vi "24-09-2020.vi"() -> ()   [LabVIEW 2020]
uses:
  <vilib>/measure/NI_MABase.lvlib
panel:
  out "reversed array":dbl[](array[numeric])
  in  "Numeric 4":dbl format="%#_13g"
  out "H":dbl
  out "D":dbl
  out "U":dbl
  in  "Numeric 3":dbl format="%#_13g"
  out "Waveform Graph 3":waveform(dbl)(graph)
  out "Numeric 2":i32
  out "numeric array":i16[](array[numeric])
  in  "Search Item":string
  in  "String":string
  in  "stop":bool
  out "Waveform Chart":dbl(graph)
  in  "Speed":dbl(slide) scale=0.0..10.0
  out "Waveform Graph 2":i32[](graph)
  out "Numeric":i32
  out "Waveform Graph":i32[](graph)
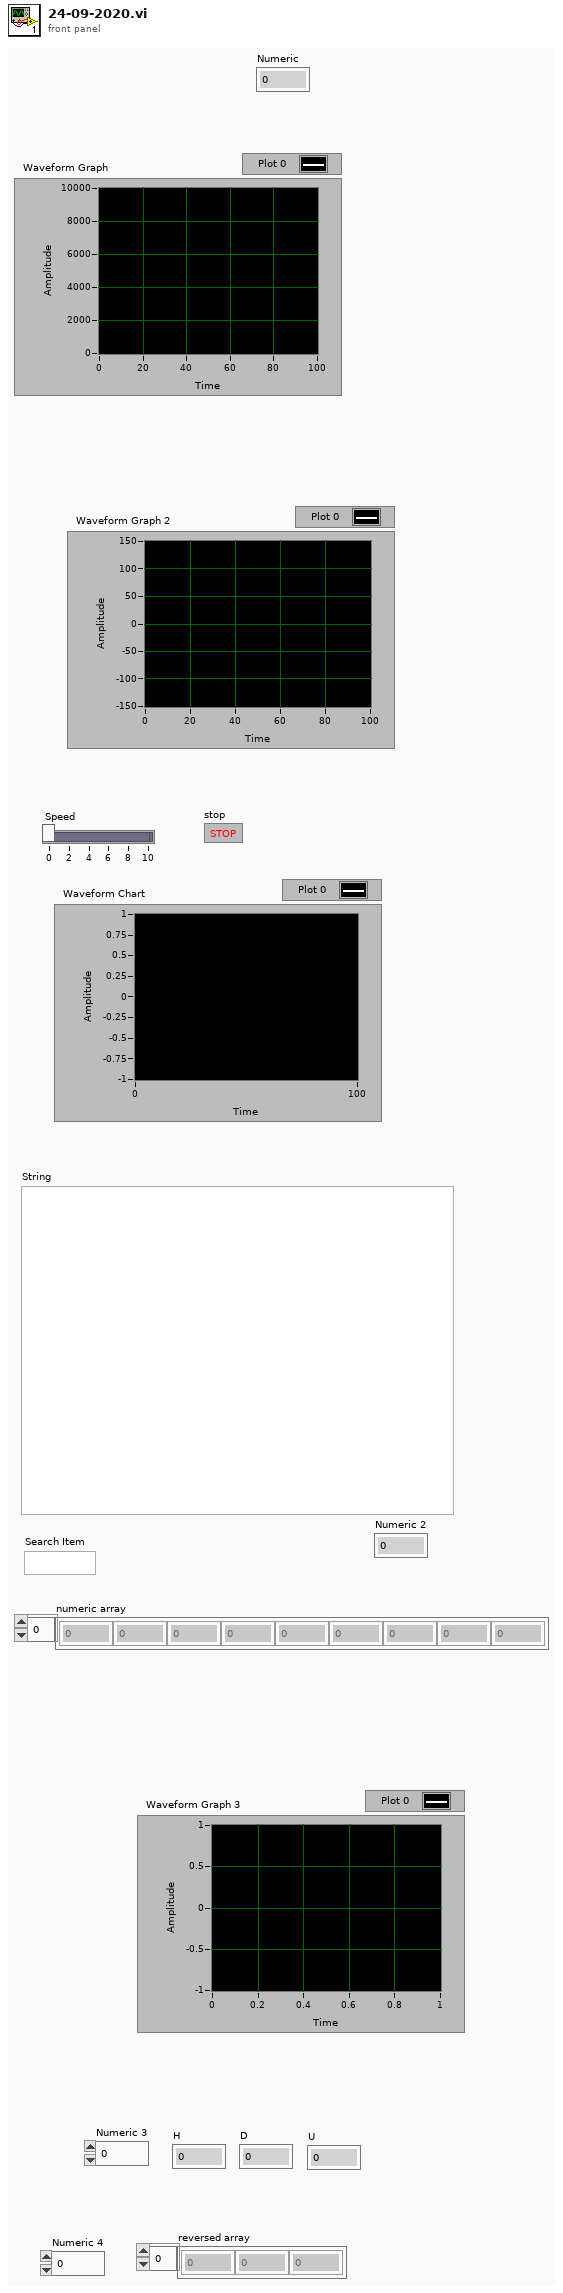
[diagram p1: front panel]
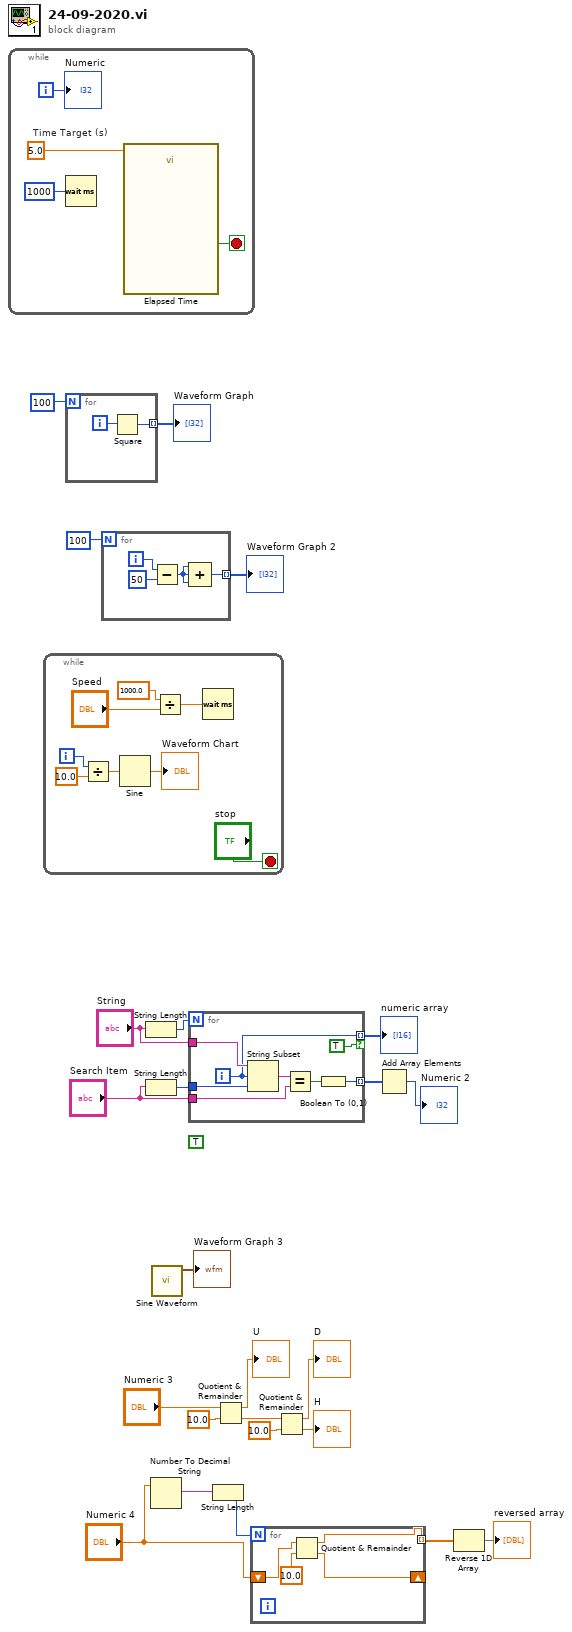
[diagram p0: block diagram]
diagram:
  (unwired) TRUE ("Boolean")
  n1 = while {
    i -> [w28]
    stop <- w26 stop-if-true
    w27 = 5.0  # Time Target (s)
    n2 = Wait (ms)(milliseconds to wait=u32 1000) -> ()  [unwired: 1 out]
    n3 = call "Elapsed Time"("Time Target (s)"=w27) -> ("Time has Elapsed"=w26:bool)  [unwired: 11 in, 7 out]
    "Numeric" <- w28
  }
  n4 = while {
    i -> [w30]
    stop <- "stop" stop-if-true
    n5 = Divide(x=w30, y=10.0 ("x")) -> (x/y=w32:dbl)
    n6 = Sine(x=w32) -> (sin(x)=→"Waveform Chart":dbl)
    n7 = Divide(x=1000.0, y="Speed") -> (x/y=w34:dbl)
    n8 = Wait (ms)(milliseconds to wait=w34) -> ()  [unwired: 1 out]
  }
  n9 = for {
    N: 100 -> [_]
    tunnel: [w37] -> w23 mode=indexing
    i -> [w38]
    n10 = Square(x=w38) -> (x^2=w37:i32)
  }
  "Waveform Graph" <- w23
  n11 = for {
    N: 100 -> [_]
    tunnel: [w39] -> w21 mode=indexing
    i -> [w41]
    n12 = Subtract(x=w41, y=50) -> (x-y=w40:i32)
    n13 = Compound Arithmetic op=ADD(w40, w40, w40) -> (w39:i32)
  }
  "Waveform Graph 2" <- w21
  n14 = String Length(string="String") -> (length=w20:i32)
  n15 = String Length(string="Search Item") -> (length=w18:i32)
  n16 = Number To Decimal String(number="Numeric 4") -> (decimal integer string=w4:string)  [unwired: 1 in]
  n17 = call <vilib>:"Sine Waveform.vi"() -> ("signal out"=→"Waveform Graph 3":waveform(dbl))  [unwired: 10 in, 1 out]
  n18 = for {
    N: w20 -> [_]
    tunnel: "String" -> [w50]
    tunnel: w18 -> [w49]
    tunnel: "Search Item" -> [w47]
    tunnel: [w46] -> w16 mode=indexing
    tunnel: [w45] -> w15 mode=indexing if=TRUE
    i -> [w45]
    n19 = String Subset(string=w50, offset (0)=w45, length (rest)=w49) -> (substring=w48:string)
    n20 = Equal?(x=w48, y=w47) -> (x = y?=w44:bool)
    n21 = Boolean To (0,1)(Boolean=w44) -> (0, 1=w46:i16)
  }
  "numeric array" <- w15
  n22 = String Length(string=w4) -> (length=w3:i32)
  n23 = Quotient & Remainder(x="Numeric 3", y=10.0) -> (x-y*floor(x/y)=→"U":dbl, floor(x/y)=w9:dbl)
  n24 = for {
    N: w3 -> [_]
    shift-right: [w51] -> _
    shift-left: "Numeric 4" -> [w54]
    tunnel: [w52] -> w2 mode=indexing
    n25 = Quotient & Remainder(x=w54, y=10.0) -> (x-y*floor(x/y)=w52:dbl, floor(x/y)=w51:dbl)
  }
  n26 = Quotient & Remainder(x=w9, y=10.0) -> (x-y*floor(x/y)=→"D":dbl, floor(x/y)=→"H":dbl)
  n27 = Add Array Elements(numeric array=w16) -> (sum=→"Numeric 2":i16)
  n28 = Reverse 1D Array(array=w2) -> (reversed array=→"reversed array":dbl[])
